vi "Message - YesNo.vi"(8 "error in":errorcluster, 11 "Message In":string="Tittle") -> (0 "error out":errorcluster, 3 "Good?":bool)   [LabVIEW 2018]
panel:
  out "Message Out":string="Tittle"
  in  "NO Button":bool
  in  "YES Button":bool
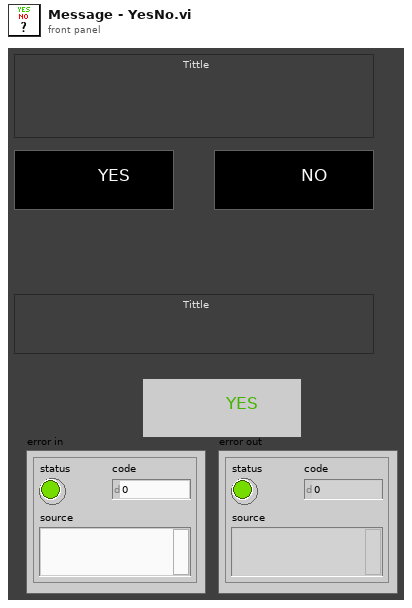
[diagram p1: front panel]
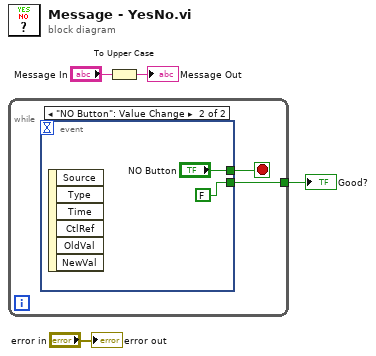
[diagram p0: block diagram]
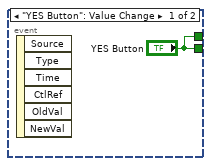
[diagram p2: hidden frame]
diagram:
  n1 = while {
    tunnel: [w5] -> w4
    stop <- w6 stop-if-true
    n2 = event shown="[1] \"NO Button\": Value Change" {
      selector: _ -> [_ _]
      dyn-events: _ -> [_ _]
      timeout: _ -> [_ _]
      tunnel: ["YES Button" "NO Button"] -> w6
      tunnel: ["YES Button" FALSE ("YES Button")] -> w5
      event "YES Button": Value Change {
        n3 = event-data() -> ()  [unwired: 1 in, 6 out]
      }
      event "NO Button": Value Change {
        n4 = event-data() -> ()  [unwired: 1 in, 6 out]
      }
    }
  }
  "Good?" <- w4
  n5 = To Upper Case(1:"Message In") -> (0:→"Message Out":string)
  "error out" <- "error in"
